vi "to_item.vi"(8 "error in (no error)":errorcluster, 11 "Table in":refnum<class "InlineTable.lvclass">) -> (0 "error out":errorcluster, 2 "Item out":refnum<class "Item.lvclass">, 3 "Table out":refnum<class "InlineTable.lvclass">)   [LabVIEW 2020, in "toml_edit.lvlib" / "InlineTable.lvclass"]
uses:
  InlineTable.lvclass
  Item/Item.lvclass
  InlineTable.lvclass/InlineTable.ctl
  dragon_toml_64.dll
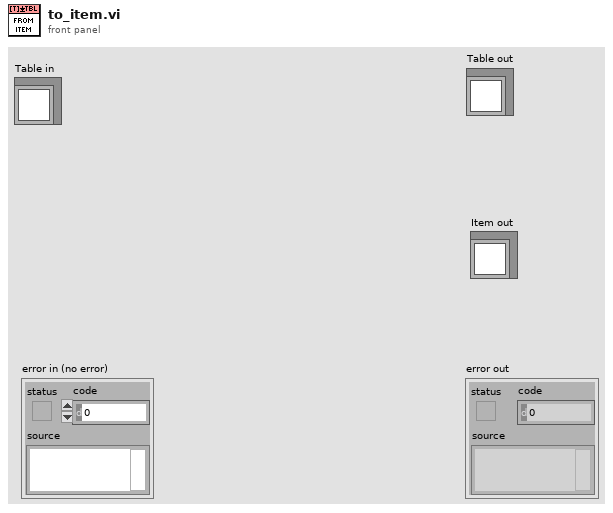
[diagram p1: front panel]
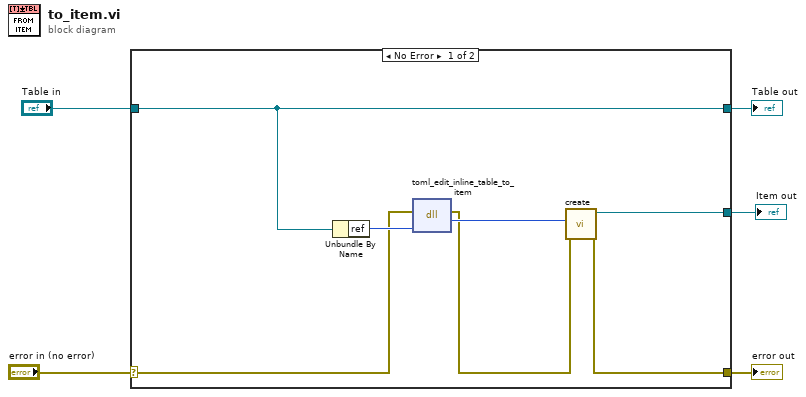
[diagram p0: block diagram]
diagram:
  n1 = case shown="No Error" "error in (no error)" {
    selector: "error in (no error)" -> [w10 w14]
    tunnel: [w6 w14] -> w4
    tunnel: [w8 w13] -> w2
    tunnel: "Table in" -> [w8 w13]
    tunnel: [w9 _] -> w1
    frame No Error {
      n2 = Unbundle By Name(w8) -> ("ref"=w11:u64)
      n3 = dll-call lib="C:/Projects/toml-edit-labview/lv_src/dragon_toml_*.dll" fn="toml_edit_inline_table_to_item"(error in=w10, "table_ref"=w11) -> (error out=w7:errorcluster, "item_ref"=w12:u64)  [unwired: 3 in, 1 out]
      n4 = call "create.vi"("error in (no error)"=w7, "ref"=w12) -> ("error out"=w6:errorcluster, "Item out"=w9:refnum<class "Item.lvclass">)  [unwired: 8 in]
    }
    frame Error {
    }
  }
  "error out" <- w4
  "Table out" <- w2
  "Item out" <- w1
